vi "Element Type.vi"(11 "ImageButtonControl in":refnum<class "ImageButtonControl.lvclass">) -> (2 "Element Type":string)   [LabVIEW 2020, in "VolatusGUIElements.lvlib" / "ImageButtonControl.lvclass"]
uses:
  ImageButtonControl.lvclass
  ImageButtonControl.lvclass/ImageButtonControl.ctl
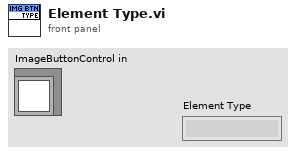
[diagram p1: front panel]
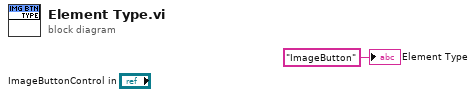
[diagram p0: block diagram]
diagram:
  "Element Type" <- "ImageButton" ("Element Type")
